vi "Parcial_Audios.vi"() -> ()   [LabVIEW 2019]
uses:
  <vilib>/Analysis/2dsp.llb/Real FFT.vi
  <vilib>/Analysis/NI_AALPro.lvlib
panel:
  out "Respuesta":string
  out "Probando":string
  out "Probando":dbl[](graph)
  out "Array":string[](array[string])
  out "Audio sonando":string
  out "Transformada":dbl[](graph)
  out "Original":waveform(dbl)(graph)
  out "4 gallina":bool
  out "2 cabinera":bool
  out "3 colibri":bool
  out "1 andigena":bool
  in  "Oir":bool
  in  "stop":bool
  in  "Enum":T1(ring)
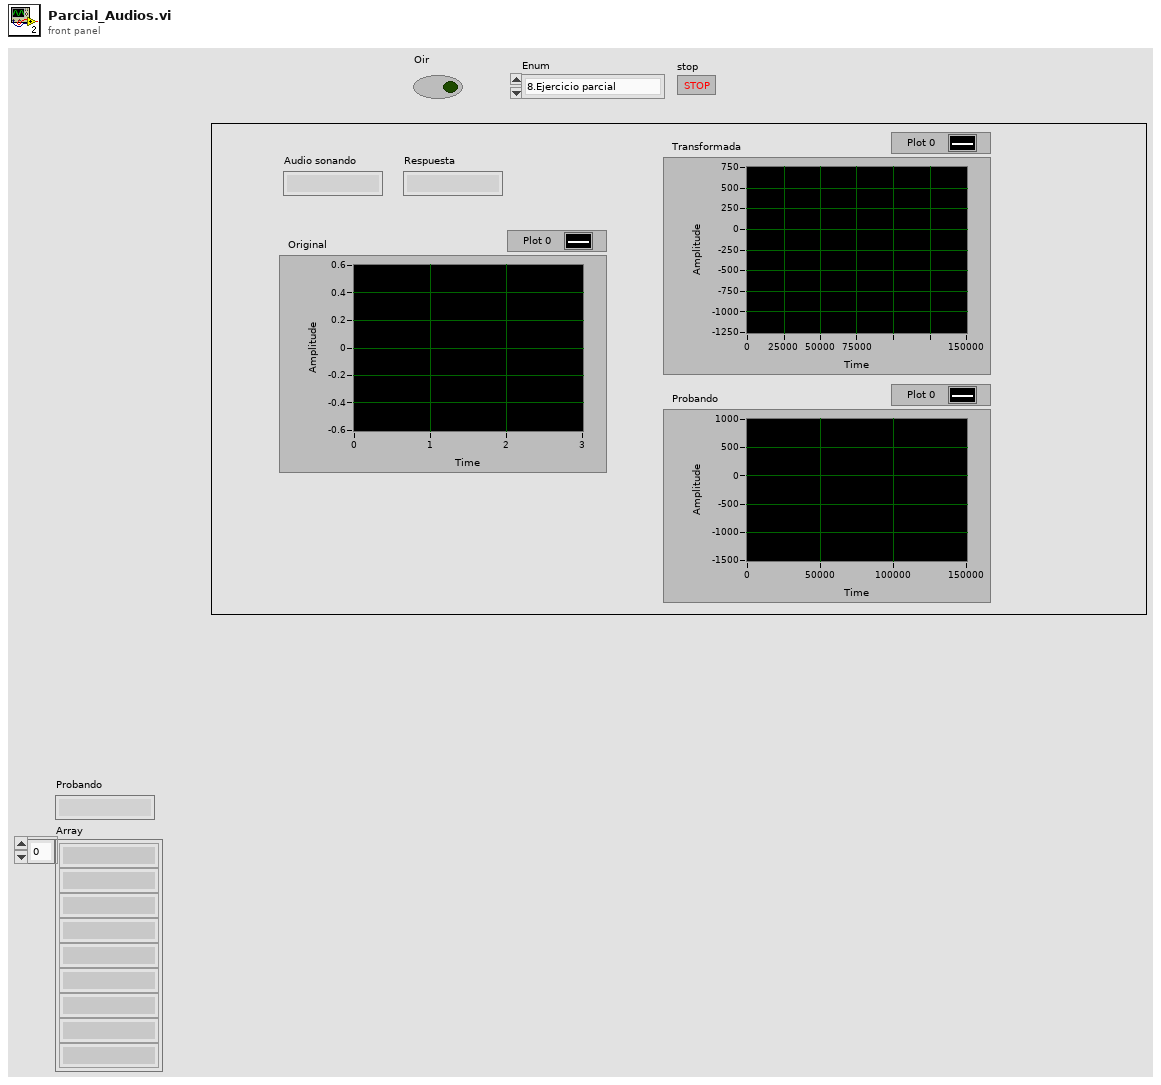
[diagram p1: front panel]
types:
  T1 = enum16{"8.Ejercicio parcial", "5.Wilmer Arias", "6.Erika ", "7.Juan Diego", "1.Andigena_nigrirostris", "2.Caminera_rabiblanca", "3.Colibri_rutilante", "4.Gallina_ciega"}
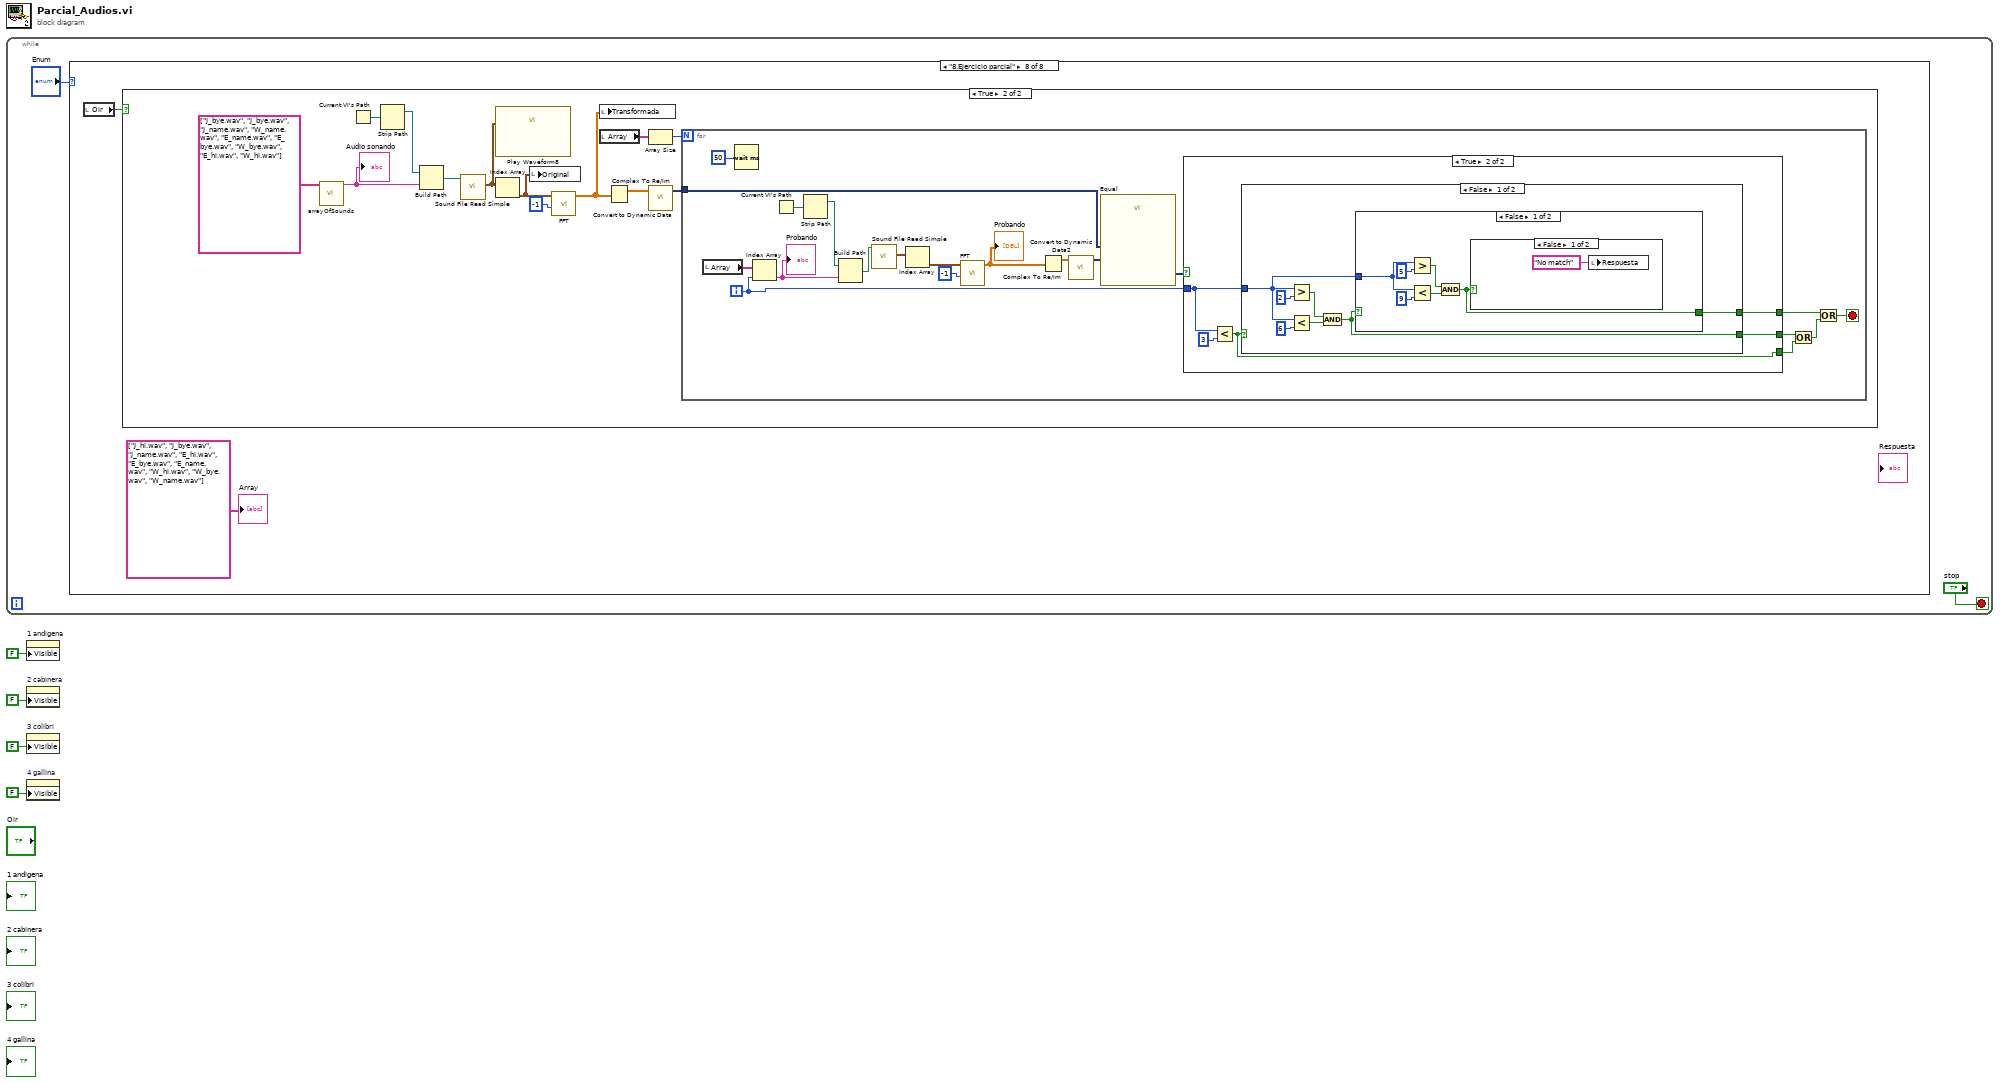
[diagram p0: block diagram]
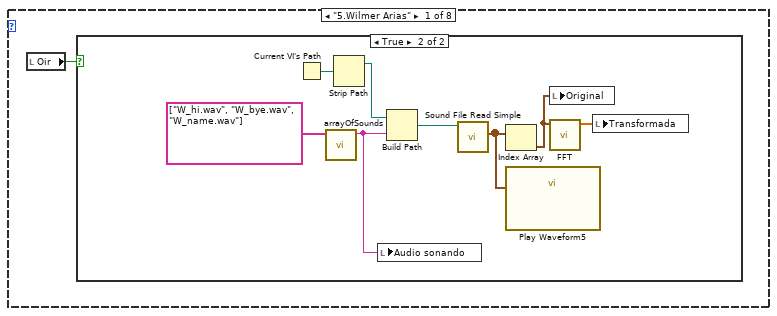
[diagram p2: hidden frame]
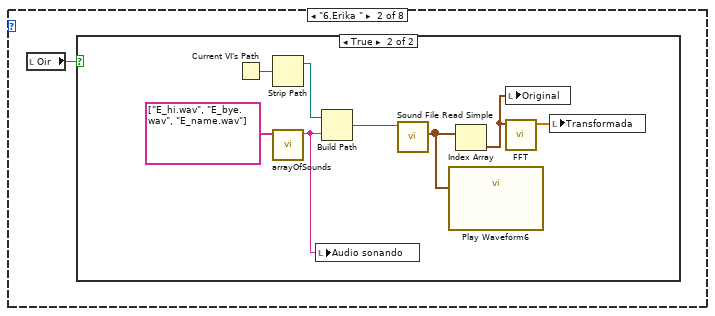
[diagram p4: hidden frame]
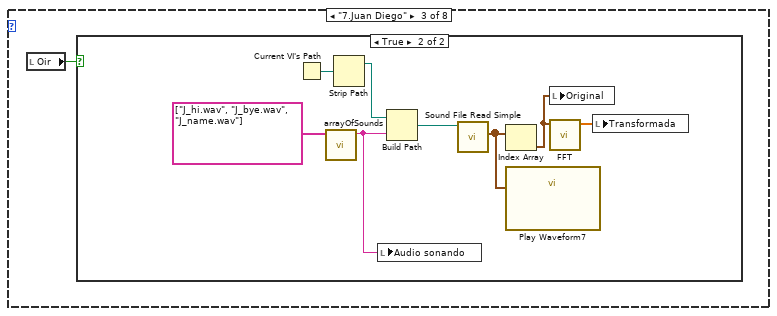
[diagram p6: hidden frame]
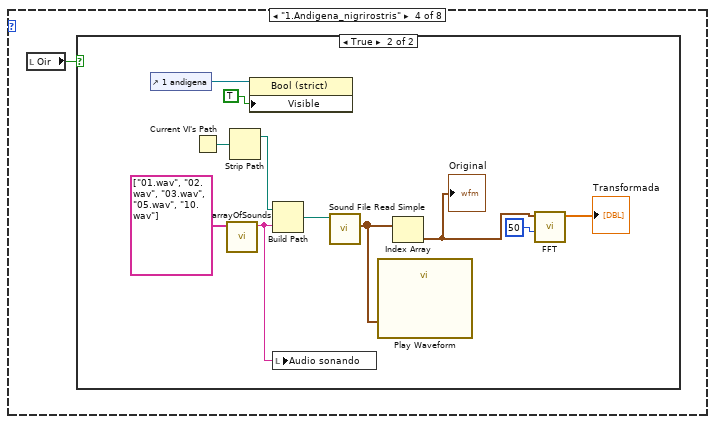
[diagram p8: hidden frame]
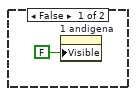
[diagram p9: hidden frame]
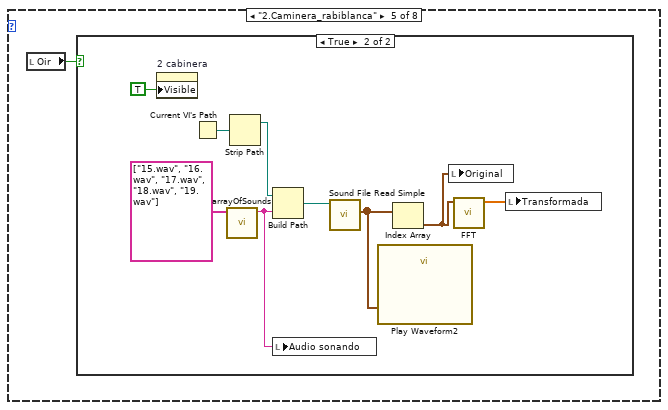
[diagram p10: hidden frame]
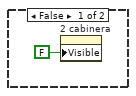
[diagram p11: hidden frame]
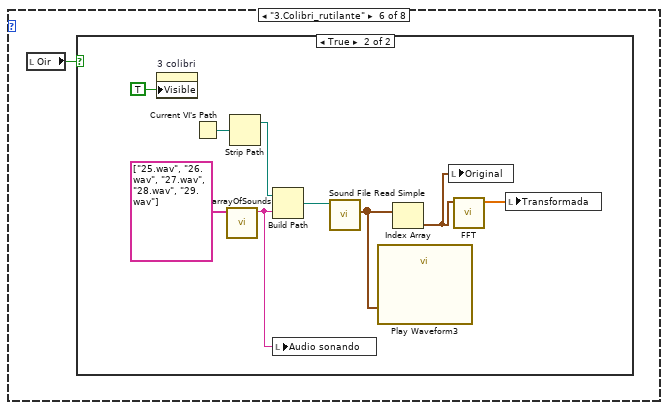
[diagram p12: hidden frame]
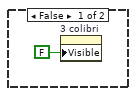
[diagram p13: hidden frame]
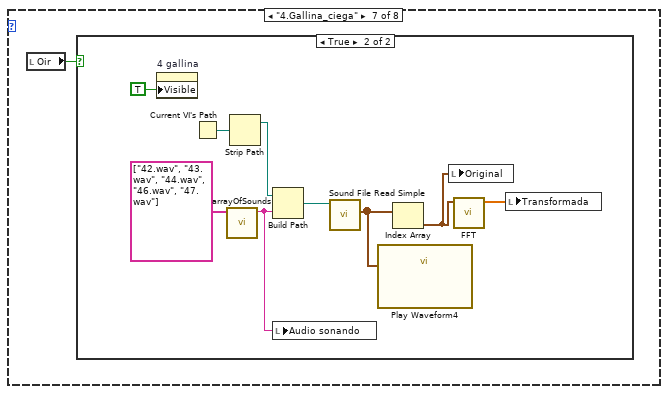
[diagram p14: hidden frame]
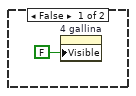
[diagram p15: hidden frame]
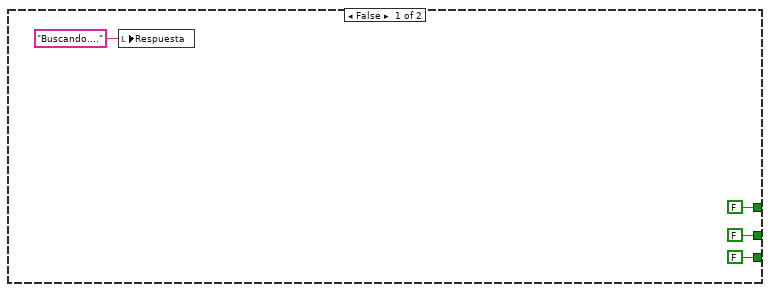
[diagram p17: hidden frame]
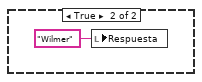
[diagram p18: hidden frame]
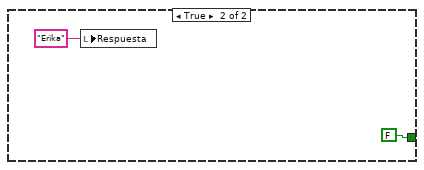
[diagram p19: hidden frame]
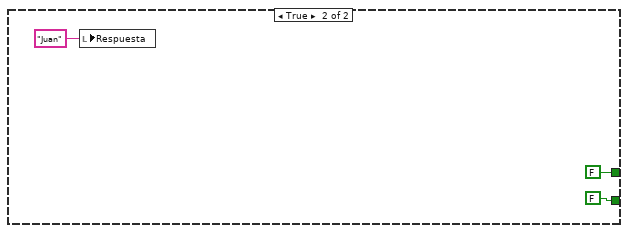
[diagram p20: hidden frame]
diagram:
  n1 = while {
    stop <- "stop" stop-if-true
    n2 = case shown="\"8.Ejercicio parcial\"" "Enum" {
      frame "5.Wilmer Arias" {
        n3 = local read "Oir"() -> (w7:bool)
        n4 = case shown="True" w7 {
          frame False {
          }
          frame True {
            n5 = Current VI's Path() -> (path=w15:path)
            n6 = call "arrayOfSounds.vi"("Array"=string[] ["W_hi.wav", "W_bye.wav", "W_name.wav"]) -> ("name or relative path"=w9:string)  [unwired: 10 in]
            n7 = Strip Path(path=w15) -> (stripped path=w14:path)  [unwired: 1 out]
            n8 = local write "Audio sonando"(w9) -> ()
            n9 = Build Path(base path=w14, name or relative path=w9) -> (appended path=w13:path)
            n10 = call <vilib>:"Sound File Read Simple.vi"("path"=w13) -> ("data"=w10:waveform(dbl)[])  [unwired: 7 in, 3 out]
            n11 = Index Array(array=w10) -> (element=w8:waveform(dbl))  [unwired: 1 in]
            n12 = call "Play Waveform5"("Data"=w10) -> ()  [unwired: 18 in, 1 out]
            n13 = local write "Original"(w8) -> ()
            n14 = call-poly <vilib>:"FFT.vi"("X"=w8) -> ("FFT {X}"=w11:cdb[])  [unwired: 9 in, 1 out]
            n15 = local write "Transformada"(w11) -> ()
          }
        }
      }
      frame "6.Erika " {
        n16 = local read "Oir"() -> (w16:bool)
        n17 = case shown="True" w16 {
          frame False {
          }
          frame True {
            n18 = Current VI's Path() -> (path=w24:path)
            n19 = Strip Path(path=w24) -> (stripped path=w23:path)  [unwired: 1 out]
            n20 = call "arrayOfSounds.vi"("Array"=string[] ["E_hi.wav", "E_bye.wav", "E_name.wav"]) -> ("name or relative path"=w17:string)  [unwired: 10 in]
            n21 = local write "Audio sonando"(w17) -> ()
            n22 = Build Path(base path=w23, name or relative path=w17) -> (appended path=w22:path)
            n23 = call <vilib>:"Sound File Read Simple.vi"("path"=w22) -> ("data"=w21:waveform(dbl)[])  [unwired: 7 in, 3 out]
            n24 = call "Play Waveform6"("Data"=w21) -> ()  [unwired: 18 in, 1 out]
            n25 = Index Array(array=w21) -> (element=w20:waveform(dbl))  [unwired: 1 in]
            n26 = local write "Original"(w20) -> ()
            n27 = call-poly <vilib>:"FFT.vi"("X"=w20) -> ("FFT {X}"=w19:cdb[])  [unwired: 9 in, 1 out]
            n28 = local write "Transformada"(w19) -> ()
          }
        }
      }
      frame "7.Juan Diego" {
        n29 = local read "Oir"() -> (w25:bool)
        n30 = case shown="True" w25 {
          frame False {
          }
          frame True {
            n31 = Current VI's Path() -> (path=w33:path)
            n32 = call "arrayOfSounds.vi"("Array"=string[] ["J_hi.wav", "J_bye.wav", "J_name.wav"]) -> ("name or relative path"=w26:string)  [unwired: 10 in]
            n33 = Strip Path(path=w33) -> (stripped path=w32:path)  [unwired: 1 out]
            n34 = local write "Audio sonando"(w26) -> ()
            n35 = Build Path(base path=w32, name or relative path=w26) -> (appended path=w31:path)
            n36 = call <vilib>:"Sound File Read Simple.vi"("path"=w31) -> ("data"=w30:waveform(dbl)[])  [unwired: 7 in, 3 out]
            n37 = Index Array(array=w30) -> (element=w29:waveform(dbl))  [unwired: 1 in]
            n38 = call "Play Waveform7"("Data"=w30) -> ()  [unwired: 18 in, 1 out]
            n39 = local write "Original"(w29) -> ()
            n40 = call-poly <vilib>:"FFT.vi"("X"=w29) -> ("FFT {X}"=w28:cdb[])  [unwired: 9 in, 1 out]
            n41 = local write "Transformada"(w28) -> ()
          }
        }
      }
      frame "1.Andigena_nigrirostris" {
        n42 = local read "Oir"() -> (w34:bool)
        n43 = case shown="True" w34 {
          frame False {
            n44 = property on="1 andigena" class="Bool (strict)"("Visible"=FALSE) -> ()  [unwired: 2 in, 2 out]
          }
          frame True {
            n45 = control-ref of="1 andigena"() -> (w45:refnum<vi>)
            n46 = Current VI's Path() -> (path=w41:path)
            n47 = call "arrayOfSounds.vi"("Array"=string[] ["01.wav", "02.wav", "03.wav", "05.wav", "10.wav"]) -> ("name or relative path"=w36:string)  [unwired: 10 in]
            n48 = Strip Path(path=w41) -> (stripped path=w40:path)  [unwired: 1 out]
            n49 = property on="Property Node" class="Bool (strict)"(reference=w45, "Visible"=TRUE) -> ()  [unwired: 1 in, 2 out]
            n50 = Build Path(base path=w40, name or relative path=w36) -> (appended path=w39:path)
            n51 = local write "Audio sonando"(w36) -> ()
            n52 = call <vilib>:"Sound File Read Simple.vi"("path"=w39) -> ("data"=w44:waveform(dbl)[])  [unwired: 7 in, 3 out]
            n53 = call "Play Waveform"("Data"=w44) -> ()  [unwired: 18 in, 1 out]
            n54 = Index Array(array=w44) -> (element=w43:waveform(dbl))  [unwired: 1 in]
            "Original" <- w43
            n55 = call-poly <vilib>:"FFT.vi"("FFT size"=50, "X"=w43) -> ("FFT {X}"=→"Transformada":cdb[])  [unwired: 8 in, 1 out]
          }
        }
      }
      frame "2.Caminera_rabiblanca" {
        n56 = local read "Oir"() -> (w47:bool)
        n57 = case shown="True" w47 {
          frame False {
            n58 = property on="2 cabinera" class="Bool (strict)"("Visible"=FALSE) -> ()  [unwired: 2 in, 2 out]
          }
          frame True {
            n59 = property on="2 cabinera" class="Bool (strict)"("Visible"=TRUE) -> ()  [unwired: 2 in, 2 out]
            n60 = Current VI's Path() -> (path=w56:path)
            n61 = call "arrayOfSounds.vi"("Array"=string[] ["15.wav", "16.wav", "17.wav", "18.wav", "19.wav"]) -> ("name or relative path"=w49:string)  [unwired: 10 in]
            n62 = Strip Path(path=w56) -> (stripped path=w55:path)  [unwired: 1 out]
            n63 = Build Path(base path=w55, name or relative path=w49) -> (appended path=w54:path)
            n64 = local write "Audio sonando"(w49) -> ()
            n65 = call <vilib>:"Sound File Read Simple.vi"("path"=w54) -> ("data"=w53:waveform(dbl)[])  [unwired: 7 in, 3 out]
            n66 = call "Play Waveform2"("Data"=w53) -> ()  [unwired: 18 in, 1 out]
            n67 = Index Array(array=w53) -> (element=w52:waveform(dbl))  [unwired: 1 in]
            n68 = local write "Original"(w52) -> ()
            n69 = call-poly <vilib>:"FFT.vi"("X"=w52) -> ("FFT {X}"=w51:cdb[])  [unwired: 9 in, 1 out]
            n70 = local write "Transformada"(w51) -> ()
          }
        }
      }
      frame "3.Colibri_rutilante" {
        n71 = local read "Oir"() -> (w58:bool)
        n72 = case shown="True" w58 {
          frame False {
            n73 = property on="3 colibri" class="Bool (strict)"("Visible"=FALSE) -> ()  [unwired: 2 in, 2 out]
          }
          frame True {
            n74 = property on="3 colibri" class="Bool (strict)"("Visible"=TRUE) -> ()  [unwired: 2 in, 2 out]
            n75 = Current VI's Path() -> (path=w67:path)
            n76 = call "arrayOfSounds.vi"("Array"=string[] ["25.wav", "26.wav", "27.wav", "28.wav", "29.wav"]) -> ("name or relative path"=w60:string)  [unwired: 10 in]
            n77 = Strip Path(path=w67) -> (stripped path=w66:path)  [unwired: 1 out]
            n78 = Build Path(base path=w66, name or relative path=w60) -> (appended path=w65:path)
            n79 = local write "Audio sonando"(w60) -> ()
            n80 = call <vilib>:"Sound File Read Simple.vi"("path"=w65) -> ("data"=w62:waveform(dbl)[])  [unwired: 7 in, 3 out]
            n81 = call "Play Waveform3"("Data"=w62) -> ()  [unwired: 18 in, 1 out]
            n82 = Index Array(array=w62) -> (element=w64:waveform(dbl))  [unwired: 1 in]
            n83 = local write "Original"(w64) -> ()
            n84 = call-poly <vilib>:"FFT.vi"("X"=w64) -> ("FFT {X}"=w61:cdb[])  [unwired: 9 in, 1 out]
            n85 = local write "Transformada"(w61) -> ()
          }
        }
      }
      frame "4.Gallina_ciega" {
        n86 = local read "Oir"() -> (w69:bool)
        n87 = case shown="True" w69 {
          frame False {
            n88 = property on="4 gallina" class="Bool (strict)"("Visible"=FALSE) -> ()  [unwired: 2 in, 2 out]
          }
          frame True {
            n89 = property on="4 gallina" class="Bool (strict)"("Visible"=TRUE) -> ()  [unwired: 2 in, 2 out]
            n90 = Current VI's Path() -> (path=w78:path)
            n91 = call "arrayOfSounds.vi"("Array"=string[] ["42.wav", "43.wav", "44.wav", "46.wav", "47.wav"]) -> ("name or relative path"=w71:string)  [unwired: 10 in]
            n92 = Strip Path(path=w78) -> (stripped path=w77:path)  [unwired: 1 out]
            n93 = Build Path(base path=w77, name or relative path=w71) -> (appended path=w76:path)
            n94 = local write "Audio sonando"(w71) -> ()
            n95 = call <vilib>:"Sound File Read Simple.vi"("path"=w76) -> ("data"=w75:waveform(dbl)[])  [unwired: 7 in, 3 out]
            n96 = call "Play Waveform4"("Data"=w75) -> ()  [unwired: 18 in, 1 out]
            n97 = Index Array(array=w75) -> (element=w74:waveform(dbl))  [unwired: 1 in]
            n98 = local write "Original"(w74) -> ()
            n99 = call-poly <vilib>:"FFT.vi"("X"=w74) -> ("FFT {X}"=w73:cdb[])  [unwired: 9 in, 1 out]
            n100 = local write "Transformada"(w73) -> ()
          }
        }
      }
      frame "8.Ejercicio parcial" {
        n101 = local read "Oir"() -> (w81:bool)
        n102 = case shown="True" w81 {
          frame False {
          }
          frame True {
            n103 = call "arrayOfSounds.vi"("Array"=string[] ["J_bye.wav", "J_bye.wav", "J_name.wav", "W_name.wav", "E_name.wav", "E_bye.wav", "W_bye.wav", "E_hi.wav", "W_hi.wav"]) -> ("name or relative path"=w90:string)  [unwired: 10 in]
            "Audio sonando" <- w90
            n104 = Current VI's Path() -> (path=w94:path)
            n105 = Strip Path(path=w94) -> (stripped path=w93:path)  [unwired: 1 out]
            n106 = Build Path(base path=w93, name or relative path=w90) -> (appended path=w92:path)
            n107 = call <vilib>:"Sound File Read Simple.vi"("path"=w92) -> ("data"=w87:waveform(dbl)[])  [unwired: 7 in, 3 out]
            n108 = call "Play Waveform8"("Data"=w87) -> ()  [unwired: 18 in, 1 out]
            n109 = Index Array(array=w87) -> (element=w88:waveform(dbl))  [unwired: 1 in]
            n110 = local write "Original"(w88) -> ()
            n111 = call-poly <vilib>:"FFT.vi"("FFT size"=-1, "X"=w88) -> ("FFT {X}"=w86:cdb[])  [unwired: 8 in, 1 out]
            n112 = local write "Transformada"(w86) -> ()
            n113 = local read "Array"() -> (w84:string[])
            n114 = Complex To Re/Im(x + iy=w86) -> (x=w85:dbl[])  [unwired: 1 out]
            n115 = Array Size(array=w84) -> (size(s)=w83:i32)
            n116 = call "Convert to Dynamic Data"("Array"=w85) -> ("Dynamic Data Type"=w82:dynamicdata)  [unwired: 3 in]
            n117 = for {
              N: w83 -> [_]
              tunnel: w82 -> [w104]
              i -> [w100]
              stop <- w95 stop-if-true
              n118 = local read "Array"() -> (w113:string[])
              n119 = Wait (ms)(milliseconds to wait=u32 50) -> ()  [unwired: 1 out]
              n120 = Index Array(array=w113, index=w100) -> (element=w106:string)
              "Probando" <- w106
              n121 = Current VI's Path() -> (path=w112:path)
              n122 = Strip Path(path=w112) -> (stripped path=w111:path)  [unwired: 1 out]
              n123 = Build Path(base path=w111, name or relative path=w106) -> (appended path=w110:path)
              n124 = call <vilib>:"Sound File Read Simple.vi"("path"=w110) -> ("data"=w109:waveform(dbl)[])  [unwired: 7 in, 3 out]
              n125 = Index Array(array=w109) -> (element=w108:waveform(dbl))  [unwired: 1 in]
              n126 = call-poly <vilib>:"FFT.vi"("FFT size"=-1, "X"=w108) -> ("FFT {X}"=w107:cdb[])  [unwired: 8 in, 1 out]
              "Probando" <- w107
              n127 = Complex To Re/Im(x + iy=w107) -> (x=w103:dbl[])  [unwired: 1 out]
              n128 = call "Convert to Dynamic Data2"("Array"=w103) -> ("Dynamic Data Type"=w102:dynamicdata)  [unwired: 3 in]
              n129 = call "Equal"("Operand 2"=w102, "Operand 1"=w104) -> ("Result"=w101:dynamicdata)  [unwired: 8 in, 1 out]
              n130 = case shown="True" w101 {
                tunnel: w100 -> [_ w122]
                tunnel: [FALSE w121] -> w99
                tunnel: [FALSE w120] -> w98
                tunnel: [FALSE w119] -> w96
                frame False {
                  n131 = local write "Respuesta"("Buscando...." ("Respuesta")) -> ()
                }
                frame True {
                  n132 = Less?(x=w122, y=3) -> (x < y?=w121:bool)
                  n133 = case shown="False" w121 {
                    tunnel: w122 -> [w125 _]
                    tunnel: [w126 FALSE] -> w120
                    tunnel: [w124 FALSE] -> w119
                    frame False {
                      n134 = Greater?(x=w125, y=2) -> (0:w127:bool)
                      n135 = Less?(x=w125, y=6) -> (x < y?=w129:bool)
                      n136 = And(x=w127, y=w129) -> (x .and. y?=w126:bool)
                      n137 = case shown="False" w126 {
                        tunnel: w125 -> [w132 _]
                        tunnel: [w133 FALSE] -> w124
                        frame False {
                          n138 = Greater?(x=w132, y=5) -> (0:w134:bool)
                          n139 = Less?(x=w132, y=9) -> (x < y?=w135:bool)
                          n140 = And(x=w134, y=w135) -> (x .and. y?=w133:bool)
                          n141 = case shown="False" w133 {
                            frame False {
                              n142 = local write "Respuesta"("No match" ("Respuesta")) -> ()
                            }
                            frame True {
                              n143 = local write "Respuesta"("Wilmer" ("Respuesta")) -> ()
                            }
                          }
                        }
                        frame True {
                          n144 = local write "Respuesta"("Erika" ("Respuesta")) -> ()
                        }
                      }
                    }
                    frame True {
                      n145 = local write "Respuesta"("Juan" ("Respuesta")) -> ()
                    }
                  }
                }
              }
              n146 = Or(x=w98, y=w99) -> (x .or. y?=w97:bool)
              n147 = Or(x=w96, y=w97) -> (x .or. y?=w95:bool)
            }
          }
        }
        "Array" <- string[] ["J_hi.wav", "J_bye.wav", "J_name.wav", "E_hi.wav", "E_bye.wav", "E_name.wav", "W_hi.wav", "W_bye.wav", "W_name.wav"]
      }
    }
  }
  n148 = property on="1 andigena" class="Bool (strict)"("Visible"=FALSE) -> ()  [unwired: 2 in, 2 out]
  n149 = property on="2 cabinera" class="Bool (strict)"("Visible"=FALSE) -> ()  [unwired: 2 in, 2 out]
  n150 = property on="3 colibri" class="Bool (strict)"("Visible"=FALSE) -> ()  [unwired: 2 in, 2 out]
  n151 = property on="4 gallina" class="Bool (strict)"("Visible"=FALSE) -> ()  [unwired: 2 in, 2 out]
